vi "CRefLabel Get Reference Index.vi"(8 "Checksum":u32, 10 "(new) Type":T1=enum."I32") -> (5 "Created":bool, 11 "Address":i32)   [LabVIEW 2012, in "CRef.lvlib"]
uses:
  CRef.lvlib
  Core/Master Types.ctl
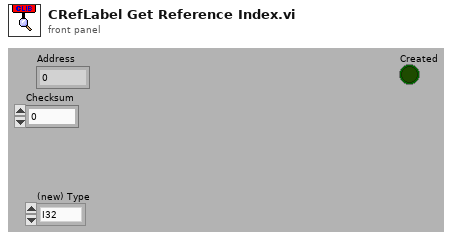
[diagram p1: front panel]
types:
  T1 = typedef "CRef.lvlib/Master Types.ctl" = enum8{"Null", "Boolean", "U8", "I8", "U16", "I16", "U32", "I32", "U64", "I64", "Single", "Double", "Extended", "CSG", "CDB", "CXT", "Boolean(Def)", "U8(Def)", "I8(Def)", "U16(Def)", "I16(Def)", "U32(Def)", "I32(Def)", "Reserved Def", "Reserved Def1", "Single(Def)", "Double(Def)", "Reserved Def2", "Reserved Def3", "Reserved Def4", "Reserved Def5", "Unsigned(Def)", "Signed(Def)", "Real(Def)", "Reserved Def6", "Numeric(Def)", "String"}
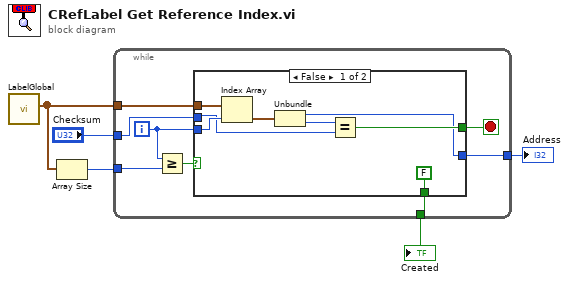
[diagram p0: block diagram]
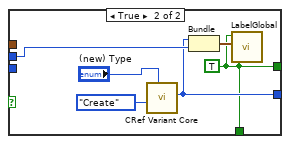
[diagram p2: hidden frame]
diagram:
  n1 = call "LabelGlobal.vi"() -> ("Lookup Table"=w2:cluster{"Address":i32, "Checksum":u32}[])  [unwired: 7 in]
  n2 = Array Size(array=w2) -> (size(s)=w5:i32)
  n3 = while {
    tunnel: w2 -> [w10]
    tunnel: w5 -> [w8]
    tunnel: [w11] -> w4
    tunnel: "Checksum" -> [w9]
    tunnel: [w6] -> w1
    i -> [w7]
    stop <- w12 stop-if-true
    n4 = Greater Or Equal?(x=w7, y=w8) -> (x >= y?=w13:bool)
    n5 = case shown="False" w13 {
      tunnel: [w19 w22] -> w12
      tunnel: w7 -> [w20 _]
      tunnel: [w15 w23] -> w11
      tunnel: w10 -> [w21 _]
      tunnel: w9 -> [w18 w25]
      tunnel: [FALSE w22] -> w6
      frame False {
        n6 = Index Array(array=w21, index=w20) -> (element=w17:cluster{"Address":i32, "Checksum":u32})
        n7 = Unbundle(w17) -> ("Address"=w15:i32, "Checksum"=w16:u32)
        n8 = Equal?(x=w16, y=w18) -> (x = y?=w19:bool)
      }
      frame True {
        w22 = TRUE
        n9 = call "CRef Variant Core.vi"("Type"="(new) Type", "Operation"=enum16{"Create", "Read", "Write", "Release"}."Create") -> ("Index"=w23:u16)  [unwired: 8 in, 1 out]
        n10 = Bundle("Index"=w23, "Checksum"=w25) -> (w24:cluster{"Index":u16, "Checksum":u32})  [unwired: 1 in]
        n11 = call "LabelGlobal.vi"("New Element"=w24, "Add"=w22) -> ()  [unwired: 5 in, 1 out]
      }
    }
  }
  "Address" <- w4
  "Created" <- w1
